vi "Test Comm L2.vi"() -> ()   [LabVIEW 2021]
uses:
  CIFChannels/Typedef/Direction.ctl
  CIF_CIPC_L2Enet.lvclass
  D:/dev/Packages/CIF_Channels_Core/src/CIPC_Channels/CIF_CIPC_Chan/CIF_CIPC_Chn.lvclass
  D:/dev/Packages/CIF_Channels_Core/src/CIFChannels/CIFChannels.lvclass
  ChannelCommon/typedef/FIFO Config.ctl
  ChannelCommon/typedef/TimeStamps.ctl
  CIF_CIPC_Chan/CIF_CIPC_Chn.lvclass/CIF_CIPC_Chn.ctl
  CIFChannels/CIFChannels.lvclass/CIFChannels.ctl
  <vilib>/CIF Foundation/CIF Utilities/DataTypes/Flatten Unflatten/Flatten U64.vi
  CIF_CIPC_Chan/SubVIs/Flatten Buffer Configuration.vi
  <vilib>/CIF Foundation/CIF Utilities/DataTypes/Flatten Unflatten/Flatten U32.vi
  <vilib>/CIF Foundation/CIF Utilities/DataTypes/Flatten Unflatten/Flatten I32.vi
  ChannelCommon/ChannelCommon.lvlib
  CIFChannels/CIFChannels.lvclass
  CIF_CIPC_Chan/CIF_CIPC_Chn.lvclass
panel:
  out "status":string
  out "pass":bool
  out "error out":errorcluster
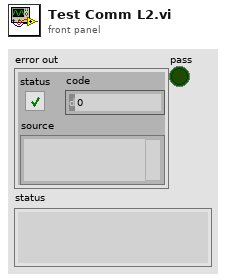
[diagram p1: front panel]
types:
  T1 = typedef "CIFChannels.lvclass/Direction.ctl" = enum16{"Publisher", "Subscriber"}
  T2 = typedef "ChannelCommon.lvlib/TimeStamps.ctl" = cluster{"ClockID":u8, "T0":i64, "T_Out":i64}
  T3 = typedef "ChannelCommon.lvlib/FIFO Config.ctl" = cluster{"Max Bytes/Msg":u64, "Max Msg/FIFO":u64, "Flags":u64}
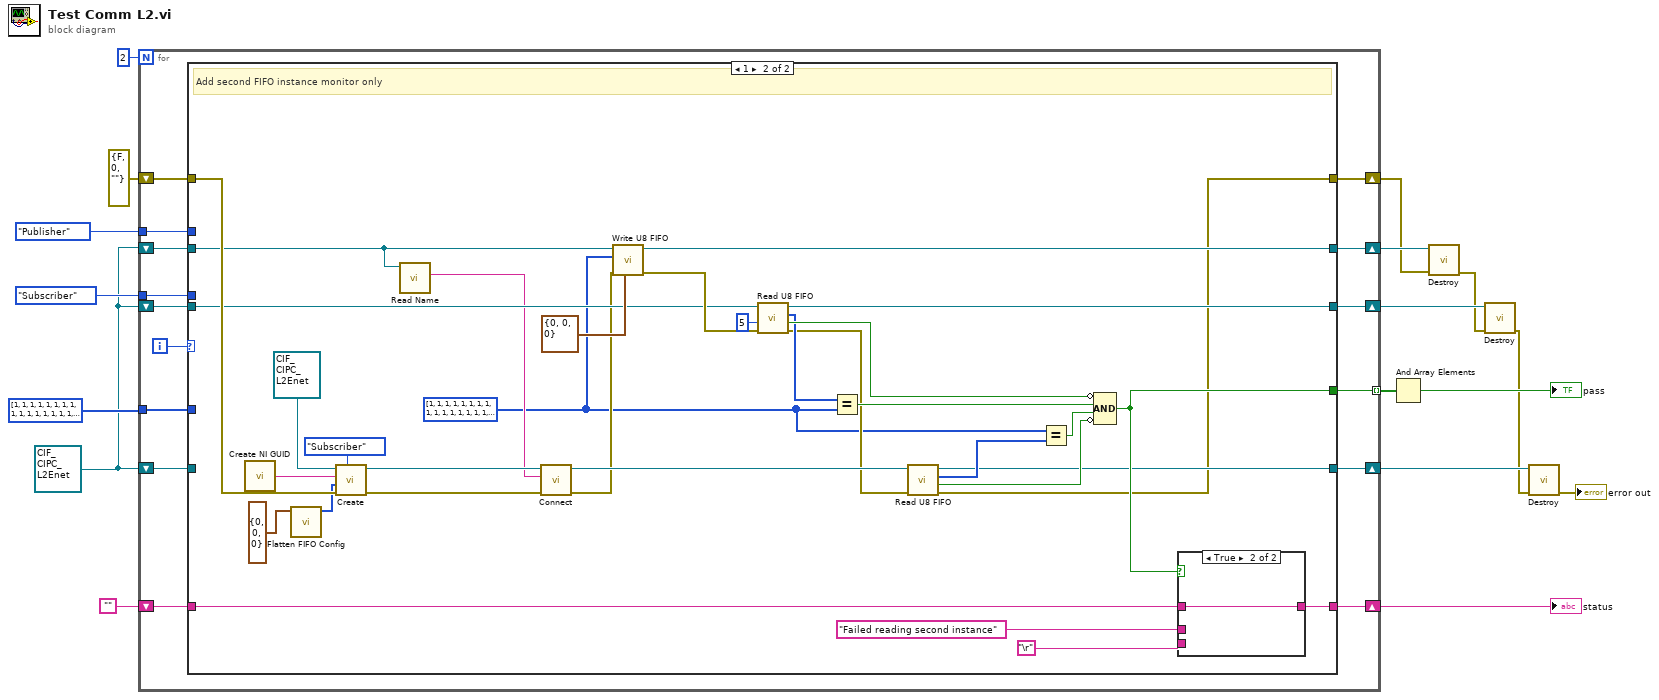
[diagram p0: block diagram]
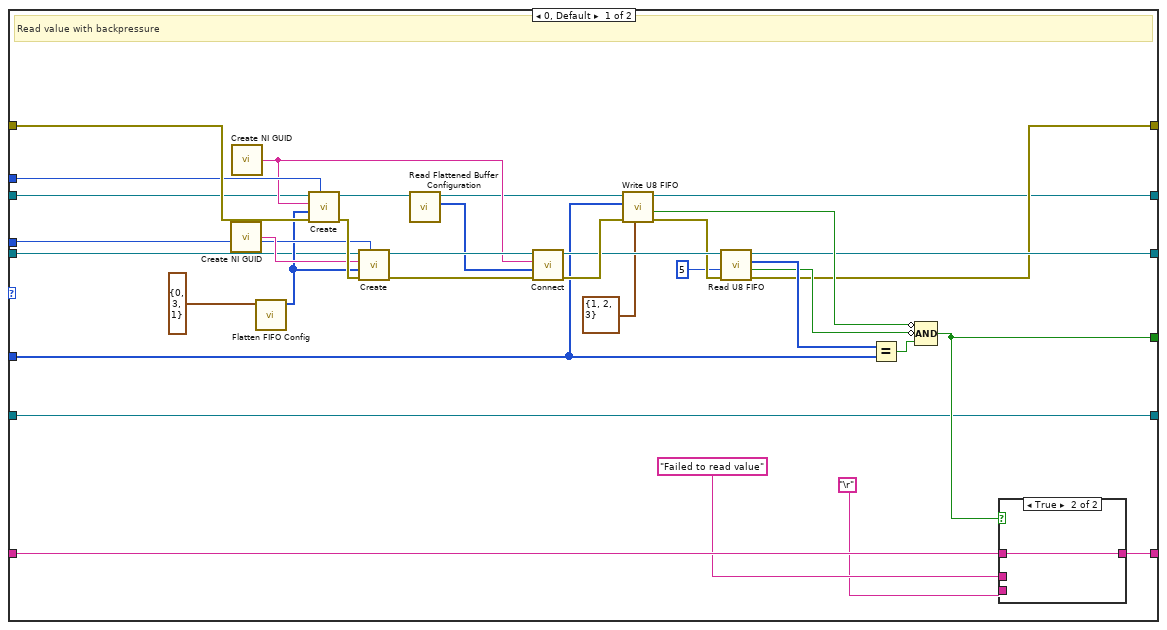
[diagram p2: hidden frame]
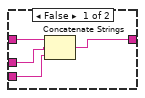
[diagram p3: hidden frame]
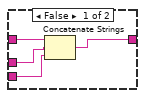
[diagram p4: hidden frame]
diagram:
  w1 = refnum<class "CIF_CIPC_L2Enet.lvclass"> refnum ("CIF_DAQ_DVR_Multi.lvclass")
  n1 = for {
    N: 2 -> [_]
    tunnel: [w32] -> w17 mode=indexing
    shift-right: [w25] -> w7
    shift-left: errorcluster {"status"=FALSE, "code"=0, "source"=""} ("error out") -> [w31]
    shift-right: [w28] -> w13
    shift-left: "" -> [w29]
    tunnel: Direction."Subscriber" ("Direction") -> [w27]
    tunnel: Direction."Publisher" ("Direction") -> [w26]
    shift-right: [w20] -> w9
    shift-left: w1 -> [w24]
    shift-right: [w19] -> w8
    shift-left: w1 -> [w18]
    tunnel: u8[] [1, 1, 1, 1, 1, 1, 1, 1, 1, 1, 1, 1, 1, 1, 1, 1, 1, 1, 1, 1, 1, 1, 1, 1, 1, 1, 1, 1, 1, 1, 1, 1, 1, 1, 1, 1, 1, 1, 1, 1, 1, 1, 1, 1, 1, 1, 1, 1, 1, 1, 1, 1, 1, 1, 1, 1, 1, 1, 1, 1, 1, 1, 1, 1, 1, 1, 1, 1, 1, 1, 1, 1, 1, 1, 1, 1, 1, 1, 1, 1, 1, 1, 1, 1, 1, 1, 1, 1, 1, 1, 1, 1, 1, 1, 1, 1, 1, 1, 1, 1, 1, 1, 1, 1, 1, 1, 1, 1, 1, 1, 1, 1, 1, 1, 1, 1, 1, 1, 1, 1, 1, 1, 1, 1, 1, 1, 1, 1, 1, 1, 1, 1, 1, 1, 1, 1, 1, 1, 1, 1, 1, 1, 1, 1, 1, 1, 1, 1, 1, 1, 1, 1, 1, 1, 1, 1, 1, 1, 1, 1, 1, 1, 1, 1, 1, 1, 1, 1, 1, 1, 1, 1, 1, 1, 1, 1, 1, 1, 1, 1, 1, 1, 1, 1, 1, 1, 1, 1, 1, 1, 1, 1, 1, 1, 1, 1, 1, 1, 1, 1, 1, 1, 1, 1, 1, 1, 1, 1, 1, 1, 1, 1, 1, 1, 1, 1, 1, 1, 1, 1, 1, 1, 1, 1, 1, 1, 1, 1, 1, 1, 1, 1, 1, 1, 1, 1, 1, 1, 1, 1, 1, 1, 1, 1, 1, 1, 1, 1, 1, 1, 1, 1, 1, 1, 1, 1, 1, 1, 1, 1, 1, 1, 1, 1, 1, 1, 1, 1, 1, 1, 1, 1, 1, 1, 1, 1, 1, 1, 1, 1, 1, 1, 1, 1, 1, 1, 1, 1, 1, 1, 1, 1, 1, 1, 1, 1, 1, 1, 1, 1, 1, 1, 1, 1, 1, 1, 1, 1, 1, 1, 1, 1, 1, 1, 1, 1, 1, 1, 1, 1, 1, 1, 1, 1, 1, 1, 1, 1, 1, 1, 1, 1, 1, 1, 1, 1, 1, 1, 1, 1, 1, 1, 1, 1, 1, 1, 1, 1, 1, 1, 1, 1, 1, 1, 1, 1, 1, 1, 1, 1, 1, 1, 1, 1, 1, 1, 1, 1, 1, 1, 1, 1, 1, 1, 1, 1, 1, 1, 1, 1, 1, 1, 1, 1, 1, 1, 1, 1, 1, 1, 1, 1, 1, 1, 1, 1, 1, 1, 1, 1, 1, 1, 1, 1, 1, 1, 1, 1, 1, 1, 1, 1, 1, 1, 1, 1, 1, 1, 1, 1, 1, 1, 1, 1, 1, 1, 1, 1, 1, 1, 1, 1, 1, 1, 1, 1, 1, 1, 1, 1, 1, 1, 1, 1, 1, 1, 1, 1, 1, 1, 1, 1, 1, 1, 1, 1, 1, 1, 1, 1, 1, 1, 1, 1, 1, 1, 1, 1, 1, 1, 1, 1, 1, 1, 1, 1, 1, 1, 1, 1, 1, 1, 1, 1, 1, 1, 1, 1, 1, 1, 1, 1, 1, 1, 1, 1, 1, 1, 1, 1, 1, 1, 1, 1, 1, 1, 1, 1, 1, 1, 1, 1, 1, 1, 1, 1, 1, 1, 1, 1, 1, 1, 1, 1, 1, 1, 1, 1, 1, 1, 1, 1, 1, 1, 1, 1, 1, 1, 1, 1, 1, 1, 1, 1, 1, 1, 1, 1, 1, 1, 1, 1, 1, 1, 1, 1, 1, 1, 1, 1, 1, 1, 1, 1, 1, 1, 1, 1, 1, 1, 1, 1, 1, 1, 1, 1, 1, 1, 1, 1, 1, 1, 1, 1, 1, 1, 1, 1, 1, 1, 1, 1, 1, 1, 1, 1, 1, 1, 1, 1, 1, 1, 1, 1, 1, 1, 1, 1, 1, 1, 1, 1, 1, 1, 1, 1, 1, 1, 1, 1, 1, 1, 1, 1, 1, 1, 1, 1, 1, 1, 1, 1, 1, 1, 1, 1, 1, 1, 1, 1, 1, 1, 1, 1, 1, 1, 1, 1, 1, 1, 1, 1, 1, 1, 1, 1, 1, 1, 1, 1, 1, 1, 1, 1, 1, 1, 1, 1, 1, 1, 1, 1, 1, 1, 1, 1, 1, 1, 1, 1, 1, 1, 1, 1, 1, 1, 1, 1, 1, 1, 1, 1, 1, 1, 1, 1, 1, 1, 1, 1, 1, 1, 1, 1, 1, 1, 1, 1, 1, 1, 1, 1, 1, 1, 1, 1, 1, 1, 1, 1, 1, 1, 1, 1, 1, 1, 1, 1, 1, 1, 1, 1, 1, 1, 1, 1, 1, 1, 1, 1, 1, 1, 1, 1, 1, 1, 1, 1, 1, 1, 1, 1, 1, 1, 1, 1, 1, 1, 1, 1, 1, 1, 1, 1, 1, 1, 1, 1, 1, 1, 1, 1, 1, 1, 1, 1, 1, 1, 1, 1, 1, 1, 1, 1, 1, 1, 1, 1, 1, 1, 1, 1, 1, 1, 1, 1, 1, 1, 1, 1, 1, 1, 1, 1, 1, 1, 1, 1, 1, 1, 1, 1, 1, 1, 1, 1, 1, 1, 1, 1, 1, 1, 1, 1, 1, 1, 1, 1, 1, 1, 1, 1, 1, 1, 1, 1, 1, 1, 1, 1, 1, 1, 1, 1, 1, 1, 1, 1, 1, 1, 1, 1, 1, 1, 1, 1, 1, 1, 1, 1, 1, 1, 1, 1, 1, 1, 1, 1, 1, 1, 1, 1, 1, 1, 1, 1, 1, 1, 1, 1, 1, 1, 1, 1, 1, 1, 1, 1, 1, 1, 1, 1, 1, 1, 1, 1, 1, 1, 1, 1, 1, 1, 1, 1, 1, 1, 1, 1, 1, 1, 1, 1, 1, 1, 1, 1, 1, 1, 1, 1, 1, 1, 1, 1, 1, 1, 1, 1, 1, 1, 1, 1, 1, 1, 1, 1, 1, 1, 1, 1, 1, 1, 1, 1, 1, 1, 1, 1, 1, 1, 1, 1, 1, 1, 1, 1, 1, 1, 1, 1, 1, 1, 1, 1, 1, 1, 1, 1, 1, 1, 1, 1, 1, 1, 1, 1, 1, 1, 1, 1, 1, 1, 1, 1, 1, 1, 1, 1, 1, 1, 1, 1, 1, 1, 1, 1, 1, 1, 1, 1, 1, 1, 1, 1, 1, 1, 1, 1, 1, 1, 1, 1, 1, 1, 1, 1, 1, 1, 1, 1, 1, 1, 1, 1, 1, 1, 1, 1, 1, 1, 1, 1, 1, 1, 1, 1, 1, 1, 1, 1, 1, 1, 1, 1, 1, 1, 1, 1, 1, 1, 1, 1, 1, 1, 1, 1, 1, 1, 1, 1, 1, 1, 1, 1, 1, 1, 1, 1, 1, 1, 1, 1, 1, 1, 1, 1, 1, 1, 1, 1, 1, 1, 1, 1, 1, 1, 1, 1, 1, 1, 1, 1, 1, 1, 1, 1, 1, 1, 1, 1, 1, 1, 1, 1, 1, 1, 1, 1, 1, 1, 1, 1, 1, 1, 1, 1, 1, 1, 1, 1, 1, 1, 1, 1, 1, 1, 1, 1, 1, 1, 1, 1, 1, 1, 1, 1, 1, 1, 1, 1, 1, 1, 1, 1, 1, 1, 1, 1, 1, 1, 1, 1, 1, 1, 1, 1, 1, 1, 1, 1, 1, 1, 1, 1, 1, 1, 1, 1, 1, 1, 1, 1, 1, 1, 1, 1, 1, 1, 1, 1, 1, 1, 1, 1, 1, 1, 1, 1, 1, 1, 1, 1, 1, 1, 1, 1, 1, 1, 1, 1, 1] ("Data in") -> [w23]
    shift-right: [w21] -> w5
    shift-left: w1 -> [w22]
    i -> [w30]
    n2 = case shown="1" w30 {
      tunnel: [w61 w100] -> w32
      tunnel: w31 -> [w59 w90]
      tunnel: [w35 w73] -> w25
      tunnel: w29 -> [w66 w104]
      tunnel: [w65 w103] -> w28
      tunnel: w27 -> [w57 _]
      tunnel: w26 -> [w56 _]
      tunnel: [w36 w82] -> w20
      tunnel: [w33 w79] -> w19
      tunnel: w18 -> [w44 w78]
      tunnel: w24 -> [w43 w80]
      tunnel: w23 -> [w34 _]
      tunnel: w22 -> [w42 _]
      tunnel: [w42 w83] -> w21
      frame 0, Default {
        # "Read value with backpressure"
        n3 = call <vilib>:"Create NI GUID.vi"() -> ("NI GUID"=w58:string)
        n4 = call <vilib>:"Create NI GUID.vi"() -> ("NI GUID"=w45:string)
        n5 = call "Flatten FIFO Config.vi"("FIFO Config in"=T3 {"Max Bytes/Msg"=0, "Max Msg/FIFO"=3, "Flags"=1}) -> ("Flattened FIFO Config"=w53:u8[])  [unwired: 10 in]
        n6 = call-dynamic "Create.vi"("Direction"=w56, "error in (no error)"=w59, "Custom Config Data"=w53, "Name"=w45, "CIFFIFO in"=w44) -> ("error out"=w60:errorcluster, "CIFFIFO out"=w41:refnum<class "CIF_CIPC_L2Enet.lvclass">)  [unwired: 5 in]
        n7 = call-dynamic "Create.vi"("Direction"=w57, "error in (no error)"=w60, "Custom Config Data"=w53, "Name"=w58, "CIFFIFO in"=w43) -> ("error out"=w46:errorcluster, "CIFFIFO out"=w54:refnum<class "CIF_CIPC_L2Enet.lvclass">)  [unwired: 5 in]
        n8 = call "Read Flattened Buffer Configuration.vi"("CIF_CIPC_Chn in"=w41) -> ("Flattened Configuration"=w40:u8[], "CIF_CIPC_Chn out"=w39:refnum<class "CIF_CIPC_L2Enet.lvclass">)  [unwired: 8 in, 1 out]
        n9 = call-dynamic "Connect.vi"("error in (no error)"=w46, "Custom Config Data"=w40, "Connection Name"=w45, "CIFTag in"=w54) -> ("error out"=w52:errorcluster, "CIFTag out"=w50:refnum<class "CIF_CIPC_L2Enet.lvclass">)  [unwired: 6 in]
        n10 = call-dynamic "Write U8 FIFO.vi"("FIFO Timestamps"=T2 {"ClockID"=1, "T0"=2, "T_Out"=3}, "error in (no error)"=w52, "Data in"=w34, "CIFFIFO in"=w39) -> ("error out"=w47:errorcluster, "timed out?"=w51:bool, "CIFFIFO out"=w33:refnum<class "CIF_CIPC_L2Enet.lvclass">)  [unwired: 4 in, 1 out]
        n11 = call-dynamic "Read U8 FIFO.vi"("error in (no error)"=w47, "Timeout (ms)"=5, "CIFFIFO in"=w50) -> ("error out"=w35:errorcluster, "timed out?"=w48:bool, "Data out"=w49:u8[], "CIFFIFO out"=w36:refnum<class "CIF_CIPC_L2Enet.lvclass">)  [unwired: 4 in, 1 out]
        n12 = Equal?(x=w49, y=w34) -> (x = y?=w62:bool)
        n13 = Compound Arithmetic op=AND(invert w51, invert w48, w62) -> (w61:bool)
        n14 = case shown="True" w61 {
          tunnel: w66 -> [w70 w71]
          tunnel: [w67 w71] -> w65
          tunnel: "Failed to read value" -> [w69 _]
          tunnel: "\r" -> [w68 _]
          frame False {
            n15 = Concatenate Strings(w70, w69, w68) -> (w67:string)
          }
          frame True {
          }
        }
      }
      frame 1 {
        w72 = u8[] [1, 1, 1, 1, 1, 1, 1, 1, 1, 1, 1, 1, 1, 1, 1, 1, 1, 1, 1, 1, 1, 1, 1, 1, 1, 1, 1, 1, 1, 1, 1, 1, 1, 1, 1, 1, 1, 1, 1, 1, 1, 1, 1, 1, 1, 1, 1, 1, 1, 1, 1, 1, 1, 1, 1, 1, 1, 1, 1, 1, 1, 1, 1, 1, 1, 1, 1, 1, 1, 1, 1, 1, 1, 1, 1, 1, 1, 1, 1, 1, 1, 1, 1, 1, 1, 1, 1, 1, 1, 1, 1, 1, 1, 1, 1, 1, 1, 1, 1, 1, 1, 1, 1, 1, 1, 1, 1, 1, 1, 1, 1, 1, 1, 1, 1, 1, 1, 1, 1, 1, 1, 1, 1, 1, 1, 1, 1, 1, 1, 1, 1, 1, 1, 1, 1, 1, 1, 1, 1, 1, 1, 1, 1, 1, 1, 1, 1, 1, 1, 1, 1, 1, 1, 1, 1, 1, 1, 1, 1, 1, 1, 1, 1, 1, 1, 1, 1, 1, 1, 1, 1, 1, 1, 1, 1, 1, 1, 1, 1, 1, 1, 1, 1, 1, 1, 1, 1, 1, 1, 1, 1, 1, 1, 1, 1, 1, 1, 1, 1, 1, 1, 1, 1, 1, 1, 1, 1, 1, 1, 1, 1, 1, 1, 1, 1, 1, 1, 1, 1, 1, 1, 1, 1, 1, 1, 1, 1, 1, 1, 1, 1, 1, 1, 1, 1, 1, 1, 1, 1, 1, 1, 1, 1, 1, 1, 1, 1, 1, 1, 1, 1, 1, 1, 1, 1, 1, 1, 1, 1, 1, 1, 1, 1, 1, 1, 1, 1, 1, 1, 1, 1, 1, 1, 1, 1, 1, 1, 1, 1, 1, 1, 1, 1, 1, 1, 1, 1, 1, 1, 1, 1, 1, 1, 1, 1, 1, 1, 1, 1, 1, 1, 1, 1, 1, 1, 1, 1, 1, 1, 1, 1, 1, 1, 1, 1, 1, 1, 1, 1, 1, 1, 1, 1, 1, 1, 1, 1, 1, 1, 1, 1, 1, 1, 1, 1, 1, 1, 1, 1, 1, 1, 1, 1, 1, 1, 1, 1, 1, 1, 1, 1, 1, 1, 1, 1, 1, 1, 1, 1, 1, 1, 1, 1, 1, 1, 1, 1, 1, 1, 1, 1, 1, 1, 1, 1, 1, 1, 1, 1, 1, 1, 1, 1, 1, 1, 1, 1, 1, 1, 1, 1, 1, 1, 1, 1, 1, 1, 1, 1, 1, 1, 1, 1, 1, 1, 1, 1, 1, 1, 1, 1, 1, 1, 1, 1, 1, 1, 1, 1, 1, 1, 1, 1, 1, 1, 1, 1, 1, 1, 1, 1, 1, 1, 1, 1, 1, 1, 1, 1, 1, 1, 1, 1, 1, 1, 1, 1, 1, 1, 1, 1, 1, 1, 1, 1, 1, 1, 1, 1, 1, 1, 1, 1, 1, 1, 1, 1, 1, 1, 1, 1, 1, 1, 1, 1, 1, 1, 1, 1, 1, 1, 1, 1, 1, 1, 1, 1, 1, 1, 1, 1, 1, 1, 1, 1, 1, 1, 1, 1, 1, 1, 1, 1, 1, 1, 1, 1, 1, 1, 1, 1, 1, 1, 1, 1, 1, 1, 1, 1, 1, 1, 1, 1, 1, 1, 1, 1, 1, 1, 1, 1, 1, 1, 1, 1, 1, 1, 1, 1, 1, 1, 1, 1, 1, 1, 1, 1, 1, 1, 1, 1, 1, 1, 1, 1, 1, 1, 1, 1, 1, 1, 1, 1, 1, 1, 1, 1, 1, 1, 1, 1, 1, 1, 1, 1, 1, 1, 1, 1, 1, 1, 1, 1, 1, 1, 1, 1, 1, 1, 1, 1, 1, 1, 1, 1, 1, 1, 1, 1, 1, 1, 1, 1, 1, 1, 1, 1, 1, 1, 1, 1, 1, 1, 1, 1, 1, 1, 1, 1, 1, 1, 1, 1, 1, 1, 1, 1, 1, 1, 1, 1, 1, 1, 1, 1, 1, 1, 1, 1, 1, 1, 1, 1, 1, 1, 1, 1, 1, 1, 1, 1, 1, 1, 1, 1, 1, 1, 1, 1, 1, 1, 1, 1, 1, 1, 1, 1, 1, 1, 1, 1, 1, 1, 1, 1, 1, 1, 1, 1, 1, 1, 1, 1, 1, 1, 1, 1, 1, 1, 1, 1, 1, 1, 1, 1, 1, 1, 1, 1, 1, 1, 1, 1, 1, 1, 1, 1, 1, 1, 1, 1, 1, 1, 1, 1, 1, 1, 1, 1, 1, 1, 1, 1, 1, 1, 1, 1, 1, 1, 1, 1, 1, 1, 1, 1, 1, 1, 1, 1, 1, 1, 1, 1, 1, 1, 1, 1, 1, 1, 1, 1, 1, 1, 1, 1, 1, 1, 1, 1, 1, 1, 1, 1, 1, 1, 1, 1, 1, 1, 1, 1, 1, 1, 1, 1, 1, 1, 1, 1, 1, 1, 1, 1, 1, 1, 1, 1, 1, 1, 1, 1, 1, 1, 1, 1, 1, 1, 1, 1, 1, 1, 1, 1, 1, 1, 1, 1, 1, 1, 1, 1, 1, 1, 1, 1, 1, 1, 1, 1, 1, 1, 1, 1, 1, 1, 1, 1, 1, 1, 1, 1, 1, 1, 1, 1, 1, 1, 1, 1, 1, 1, 1, 1, 1, 1, 1, 1, 1, 1, 1, 1, 1, 1, 1, 1, 1, 1, 1, 1, 1, 1, 1, 1, 1, 1, 1, 1, 1, 1, 1, 1, 1, 1, 1, 1, 1, 1, 1, 1, 1, 1, 1, 1, 1, 1, 1, 1, 1, 1, 1, 1, 1, 1, 1, 1, 1, 1, 1, 1, 1, 1, 1, 1, 1, 1, 1, 1, 1, 1, 1, 1, 1, 1, 1, 1, 1, 1, 1, 1, 1, 1, 1, 1, 1, 1, 1, 1, 1, 1, 1, 1, 1, 1, 1, 1, 1, 1, 1, 1, 1, 1, 1, 1, 1, 1, 1, 1, 1, 1, 1, 1, 1, 1, 1, 1, 1, 1, 1, 1, 1, 1, 1, 1, 1, 1, 1, 1, 1, 1, 1, 1, 1, 1, 1, 1, 1, 1, 1, 1, 1, 1, 1, 1, 1, 1, 1, 1, 1, 1, 1, 1, 1, 1, 1, 1, 1, 1, 1, 1, 1, 1, 1, 1, 1, 1, 1, 1, 1, 1, 1, 1, 1, 1, 1, 1, 1, 1, 1, 1, 1, 1, 1, 1, 1, 1, 1, 1, 1, 1, 1, 1, 1, 1, 1, 1, 1, 1, 1, 1, 1, 1, 1, 1, 1, 1, 1, 1, 1, 1, 1, 1, 1, 1, 1, 1, 1, 1, 1, 1, 1, 1, 1, 1, 1, 1, 1, 1, 1, 1, 1, 1, 1, 1, 1, 1, 1, 1, 1, 1, 1, 1, 1, 1, 1, 1, 1, 1, 1, 1, 1, 1, 1, 1, 1, 1, 1, 1, 1, 1, 1, 1, 1, 1, 1, 1, 1, 1, 1, 1, 1, 1, 1, 1, 1, 1, 1, 1, 1, 1, 1, 1, 1, 1, 1, 1, 1, 1, 1, 1, 1, 1, 1, 1, 1, 1, 1, 1, 1, 1, 1, 1, 1, 1, 1, 1, 1, 1, 1, 1, 1, 1, 1, 1, 1, 1, 1, 1, 1, 1, 1, 1, 1, 1, 1, 1, 1, 1, 1, 1, 1, 1, 1, 1, 1, 1, 1, 1, 1, 1, 1, 1, 1, 1, 1, 1, 1, 1, 1, 1, 1, 1, 1, 1, 1, 1, 1, 1, 1, 1, 1, 2] ("Data in")
        # "Add second FIFO instance monitor only"
        n16 = call <vilib>:"Create NI GUID.vi"() -> ("NI GUID"=w92:string)
        n17 = call "Flatten FIFO Config.vi"("FIFO Config in"=T3 {"Max Bytes/Msg"=0, "Max Msg/FIFO"=0, "Flags"=0}) -> ("Flattened FIFO Config"=w89:u8[])  [unwired: 10 in]
        n18 = call-dynamic "Create.vi"("Direction"=Direction."Subscriber", "error in (no error)"=w90, "Custom Config Data"=w89, "Name"=w92, "CIFFIFO in"=refnum<class "CIF_CIPC_L2Enet.lvclass"> refnum ("CIF_DAQ_DVR_Multi.lvclass")) -> ("error out"=w81:errorcluster, "CIFFIFO out"=w91:refnum<class "CIF_CIPC_L2Enet.lvclass">)  [unwired: 5 in]
        n19 = call "Read Name.vi"("CIFChannels in"=w78) -> ("Name"=w77:string)  [unwired: 8 in, 2 out]
        n20 = call-dynamic "Connect.vi"("error in (no error)"=w81, "Connection Name"=w77, "CIFTag in"=w91) -> ("error out"=w75:errorcluster, "CIFTag out"=w76:refnum<class "CIF_CIPC_L2Enet.lvclass">)  [unwired: 7 in]
        n21 = call-dynamic "Write U8 FIFO.vi"("FIFO Timestamps"=T2 {"ClockID"=0, "T0"=0, "T_Out"=0}, "error in (no error)"=w75, "Data in"=w72, "CIFFIFO in"=w78) -> ("error out"=w85:errorcluster, "CIFFIFO out"=w79:refnum<class "CIF_CIPC_L2Enet.lvclass">)  [unwired: 4 in, 2 out]
        n22 = call-dynamic "Read U8 FIFO.vi"("error in (no error)"=w85, "Timeout (ms)"=5, "CIFFIFO in"=w80) -> ("error out"=w74:errorcluster, "timed out?"=w96:bool, "Data out"=w95:u8[], "CIFFIFO out"=w82:refnum<class "CIF_CIPC_L2Enet.lvclass">)  [unwired: 4 in, 1 out]
        n23 = Equal?(x=w95, y=w72) -> (x = y?=w98:bool)
        n24 = call-dynamic "Read U8 FIFO.vi"("error in (no error)"=w74, "CIFFIFO in"=w76) -> ("error out"=w73:errorcluster, "timed out?"=w84:bool, "Data out"=w86:u8[], "CIFFIFO out"=w83:refnum<class "CIF_CIPC_L2Enet.lvclass">)  [unwired: 5 in, 1 out]
        n25 = Equal?(x=w72, y=w86) -> (x = y?=w99:bool)
        n26 = Compound Arithmetic op=AND(invert w96, w98, w99, invert w84) -> (w100:bool)
        n27 = case shown="True" w100 {
          tunnel: w104 -> [w108 w109]
          tunnel: [w105 w109] -> w103
          tunnel: "Failed reading second instance" -> [w107 _]
          tunnel: "\r" -> [w106 _]
          frame False {
            n28 = Concatenate Strings(w108, w107, w106) -> (w105:string)
          }
          frame True {
          }
        }
      }
    }
  }
  "status" <- w13
  n29 = And Array Elements(Boolean array=w17) -> (logical AND=→"pass":bool)
  n30 = call-dynamic "Destroy.vi"("error in (no error)"=w7, "CIFTag in"=w8) -> ("error out"=w6:errorcluster)  [unwired: 8 in, 1 out]
  n31 = call-dynamic "Destroy.vi"("error in (no error)"=w6, "CIFTag in"=w9) -> ("error out"=w4:errorcluster)  [unwired: 8 in, 1 out]
  n32 = call-dynamic "Destroy.vi"("error in (no error)"=w4, "CIFTag in"=w5) -> ("error out"=→"error out":errorcluster)  [unwired: 8 in, 1 out]
